vi "Calculations.vi"(7 "FWHM x (px)":dbl, 8 "Calibration µm/px":dbl, 9 "Energy in 1 Pulse (mJ)":dbl, 10 "Pulse Duration (fs)":dbl, 11 "FWHM y (px)":dbl) -> (0 "FWHM y (µm)":dbl, 1 "FWHM x (µm)":dbl, 2 "Peak Power (TW)":dbl, 3 "Integral of Perfect Gaussian (x10^18 W/cm²)":dbl)   [LabVIEW 2014]
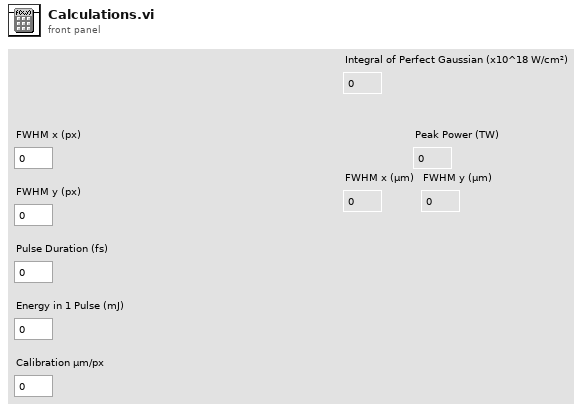
[diagram p1: front panel]
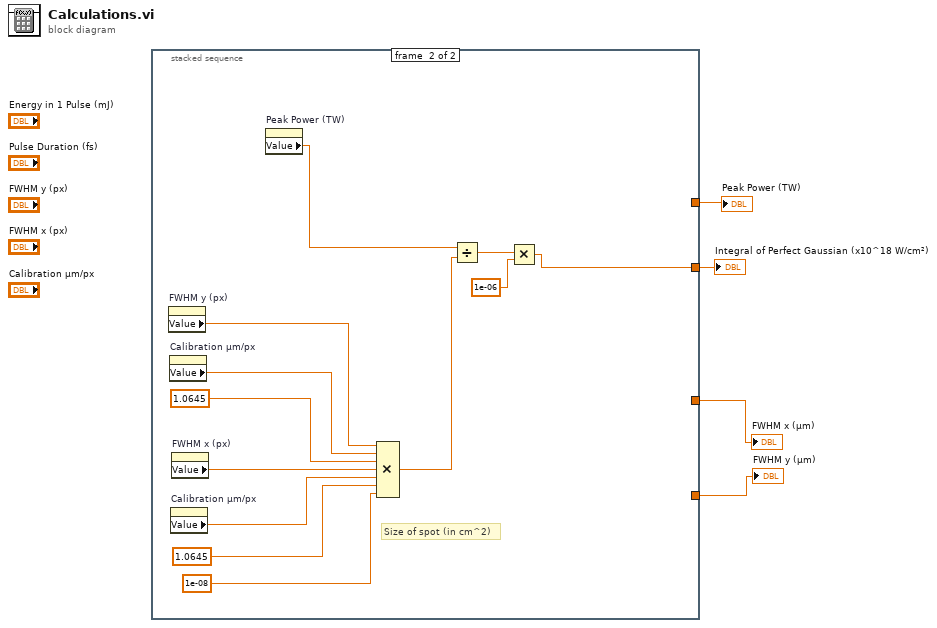
[diagram p0: block diagram]
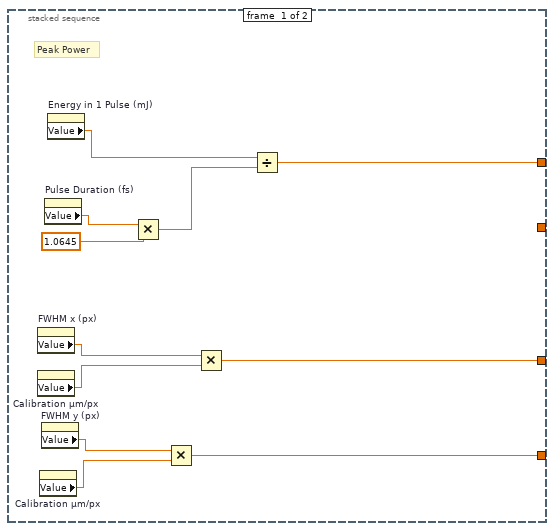
[diagram p2: hidden frame]
diagram:
  n1 = stacked-sequence {
    tunnel: [w11 _] -> w4
    tunnel: [w6 _] -> w3
    tunnel: [w5 _] -> w2
    tunnel: [_ w16] -> w1
    frame #0 {
      # "Peak Power"
      n2 = property on="FWHM x (px)" class="DigNum (strict)"() -> ("Value"=w8:dbl)  [unwired: 2 in, 2 out]
      n3 = property on="Calibration µm/px" class="DigNum (strict)"() -> ("Value"=w7:dbl)  [unwired: 2 in, 2 out]
      n4 = property on="Calibration µm/px" class="DigNum (strict)"() -> ("Value"=w9:dbl)  [unwired: 2 in, 2 out]
      n5 = property on="FWHM y (px)" class="DigNum (strict)"() -> ("Value"=w10:dbl)  [unwired: 2 in, 2 out]
      n6 = property on="Pulse Duration (fs)" class="DigNum (strict)"() -> ("Value"=w15:dbl)  [unwired: 2 in, 2 out]
      n7 = property on="Energy in 1 Pulse (mJ)" class="DigNum (strict)"() -> ("Value"=w13:dbl)  [unwired: 2 in, 2 out]
      n8 = Multiply(x=w15, y=1.0645) -> (x*y=w12:dbl)
      n9 = Multiply(x=w10, y=w9) -> (x*y=w5:dbl)
      n10 = Multiply(x=w8, y=w7) -> (x*y=w6:dbl)
      n11 = Divide(x=w13, y=w12) -> (x/y=w11:dbl)
    }
    frame #1 {
      # "Size of spot (in cm^2)"
      n12 = property on="FWHM y (px)" class="DigNum (strict)"() -> ("Value"=w25:dbl)  [unwired: 2 in, 2 out]
      n13 = property on="Calibration µm/px" class="DigNum (strict)"() -> ("Value"=w24:dbl)  [unwired: 2 in, 2 out]
      n14 = property on="Calibration µm/px" class="DigNum (strict)"() -> ("Value"=w23:dbl)  [unwired: 2 in, 2 out]
      n15 = property on="FWHM x (px)" class="DigNum (strict)"() -> ("Value"=w26:dbl)  [unwired: 2 in, 2 out]
      n16 = property on="Peak Power (TW)" class="DigNum (strict)"() -> ("Value"=w19:dbl)  [unwired: 2 in, 2 out]
      n17 = Compound Arithmetic op=MULTIPLY(w25, w24, 1.0645 ("value"), w26, w23, 1.0645 ("value"), 1e-08 ("value")) -> (w20:dbl)
      n18 = Divide(x=w19, y=w20) -> (x/y=w18:dbl)
      n19 = Multiply(x=w18, y=1e-06 ("value")) -> (x*y=w16:dbl)
    }
  }
  "Peak Power (TW)" <- w4
  "Integral of Perfect Gaussian (x10^18 W/cm²)" <- w1
  "FWHM x (µm)" <- w3
  "FWHM y (µm)" <- w2
